vi "Update Main GUI - Plot.vi"(8 "error in":errorcluster, 10 "GUI Command":T1, 11 "Main GUI Refnum":refnum<vi>) -> (0 "error out":errorcluster)   [LabVIEW 2017, in "DTacq Plot Display Library.lvlib"]
uses:
  DTacq Plot Display Library.lvlib
  Typedefs/Graphical Interface Commands - Plot--Enum.ctl
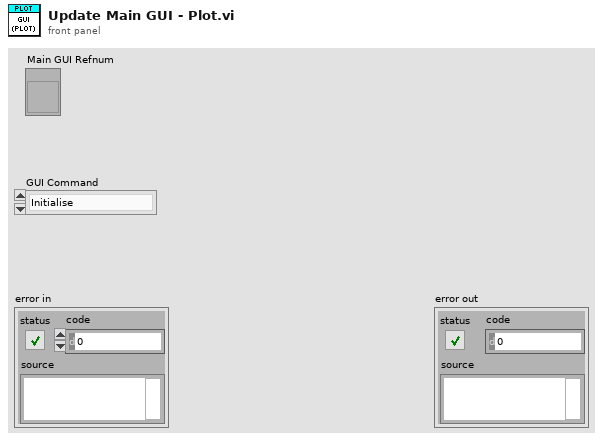
[diagram p1: front panel]
types:
  T1 = typedef "DTacq Plot Display Library.lvlib/Graphical Interface Commands - Plot--Enum.ctl" = enum16{"Initialise", "Set Plot Title"}
  T2 = typedef "LVRectTypeDef.ctl" = cluster{"Left":i16, "Top":i16, "Right":i16, "Bottom":i16}
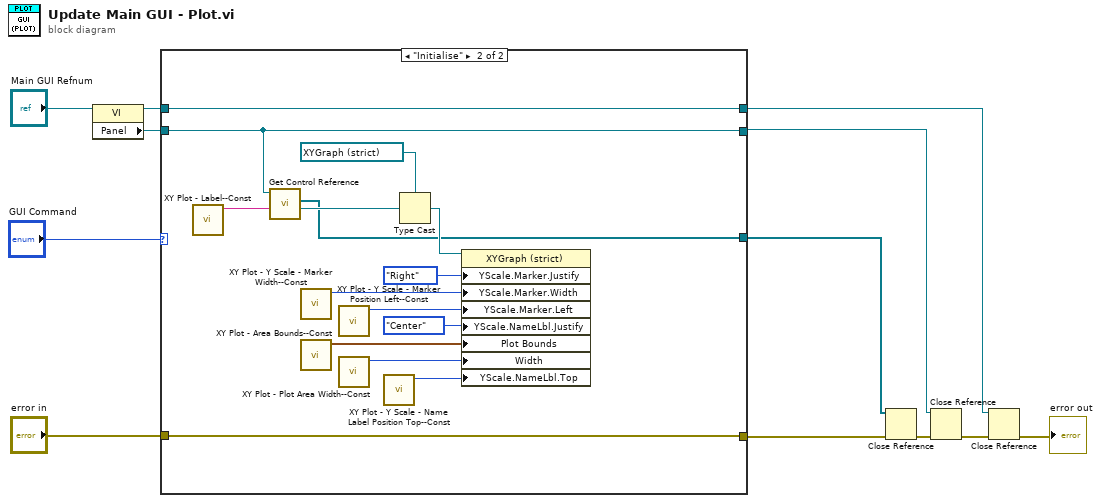
[diagram p0: block diagram]
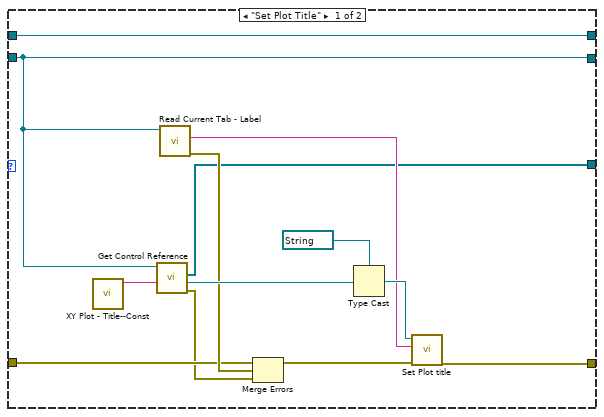
[diagram p2: hidden frame]
diagram:
  n1 = property class="VI"(reference="Main GUI Refnum") -> (reference out=w8:refnum<vi>, "Panel"=w9:refnum<vi>)  [unwired: 1 in, 1 out]
  n2 = case shown="\"Initialise\"" "GUI Command" {
    tunnel: "error in" -> [w19 w40]
    tunnel: [w17 w34] -> w11
    tunnel: [w25 w40] -> w6
    tunnel: w9 -> [w17 w34]
    tunnel: w8 -> [w16 w39]
    tunnel: [w14 w33] -> w7
    tunnel: [w16 w39] -> w2
    frame "Set Plot Title" {
      n3 = call "XY Plot - Title--Const.vi"() -> ("XY Plot Title"=w22:string)  [unwired: 11 in]
      n4 = call "Get Control Reference.vi"("Control Label"=w22, "Front Panel Reference In"=w17) -> ("error out"=w13:errorcluster, "Selected Control Reference"=w24:refnum<vi>, "Control References Array"=w14:refnum<vi>[])  [unwired: 6 in, 1 out]
      n5 = call "Read Current Tab - Label.vi"("Front Panel Reference In"=w17) -> ("error out"=w20:errorcluster, "Tab Label"=w21:string)  [unwired: 8 in, 1 out]
      n6 = Merge Errors(w19, w20, w13) -> (w18:errorcluster)
      n7 = Type Cast(type=refnum<vi> refnum ("XY Plot Title"), x=w24) -> (*(type *) &x=w23:refnum<vi>)
      n8 = call "Set Plot title.vi"("error in"=w18, "Title Text"=w21, "XY Plot Title Reference"=w23) -> ("error out"=w25:errorcluster)  [unwired: 7 in, 1 out]
    }
    frame "Initialise" {
      n9 = call "XY Plot - Label--Const.vi"() -> ("XY Plot Graph"=w38:string)  [unwired: 11 in]
      n10 = call "Get Control Reference.vi"("Control Label"=w38, "Front Panel Reference In"=w34) -> ("Selected Control Reference"=w37:refnum<vi>, "Control References Array"=w33:refnum<vi>[])  [unwired: 6 in, 2 out]
      n11 = call "XY Plot - Y Scale - Marker Width--Const.vi"() -> ("Y Scale.Marker.Size:Width"=w31:u32)  [unwired: 11 in]
      n12 = call "XY Plot - Area Bounds--Const.vi"() -> ("Plot Area Bounds"=w28:T2)  [unwired: 11 in]
      n13 = call "XY Plot - Y Scale - Marker Position Left--Const.vi"() -> ("Y Scale.Marker.Position:Left"=w30:i32)  [unwired: 11 in]
      n14 = call "XY Plot - Plot Area Width--Const.vi"() -> ("Plot Area:Size:Width"=w27:u32)  [unwired: 11 in]
      n15 = call "XY Plot - Y Scale - Name Label Position Top--Const.vi"() -> ("Y Scale.Name Label.Position:Top"=w26:i32)  [unwired: 11 in]
      n16 = Type Cast(type=refnum<vi> refnum ("reference"), x=w37) -> (*(type *) &x=w35:refnum<vi>)
      n17 = property class="XYGraph (strict)"(reference=w35, "YScale.Marker.Justify"=enum16{"Left", "Center", "Right"}."Right" ("Y Scale.Marker.Justification"), "YScale.Marker.Width"=w31, "YScale.Marker.Left"=w30, "YScale.NameLbl.Justify"=enum16{"Left", "Center", "Right"}."Center" ("Y Scale.Name Label.Justification"), "Plot Bounds"=w28, "Width"=w27, "YScale.NameLbl.Top"=w26) -> ()  [unwired: 1 in, 2 out]
    }
  }
  n18 = Close Reference(reference=w7, error in (no error)=w6) -> (error out=w5:errorcluster)
  n19 = Close Reference(reference=w11, error in (no error)=w5) -> (error out=w4:errorcluster)
  n20 = Close Reference(reference=w2, error in (no error)=w4) -> (error out=→"error out":errorcluster)
